vi "Raman_READ_WRITE.vi"(8 "error constant":errorcluster, 9 "Number of files to read":dbl=1.0, 11 "IR Read Dir.":string) -> (0 "error constant 2":errorcluster, 2 "averagePeaksStr":string, 3 "averagePeaks":dbl[](array[numeric]), 4 "Is SS?":bool)   [LabVIEW 2015]
panel:
  # "IR Data Read and Write"
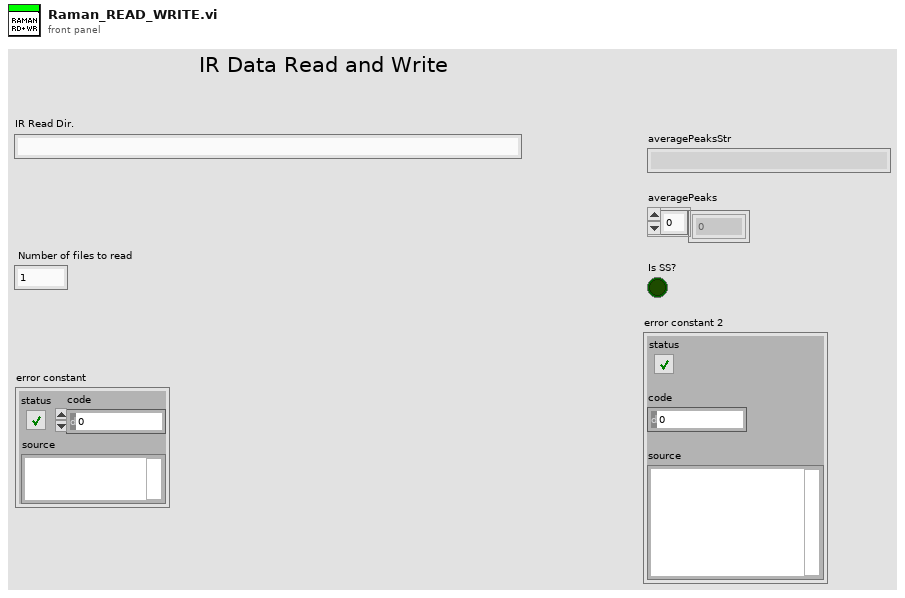
[diagram p1: front panel]
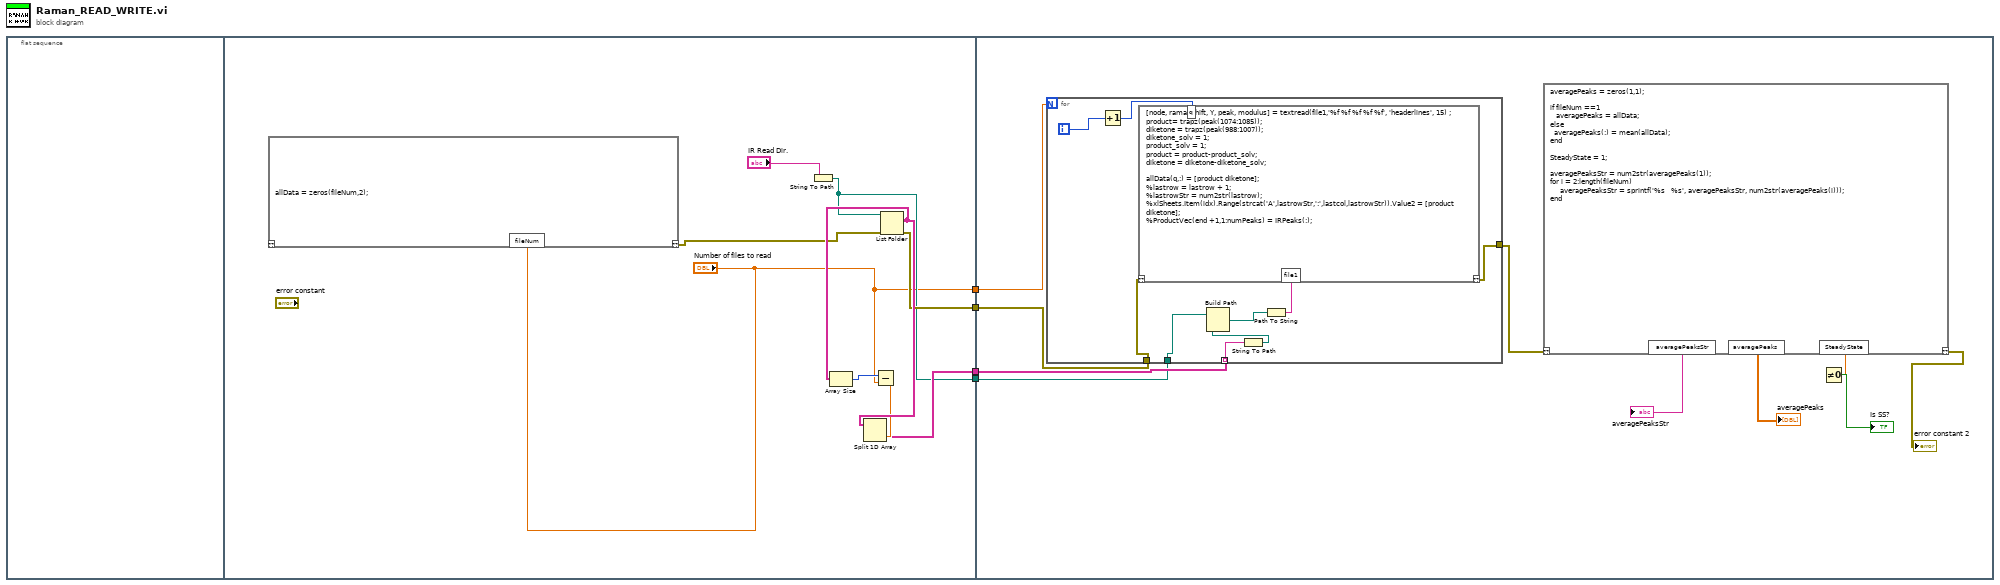
[diagram p0: block diagram]
diagram:
  n1 = flat-sequence {
    tunnel: [w8] -> w4
    tunnel: [w7] -> w3
    tunnel: [w6] -> w2
    tunnel: ["Number of files to read"] -> w1
    tunnel: w4 -> [w17]
    tunnel: w3 -> [w16]
    tunnel: w2 -> [w15]
    tunnel: w1 -> [w14]
    frame #0 {
    }
    frame #1 {
      n2 = script code="allData = zeros(fileNum,2);"("fileNum"="Number of files to read") -> ("??"=w9:errorcluster)  [unwired: 1 in]
      n3 = String To Path(string="IR Read Dir.") -> (path=w6:path)
      n4 = List Folder(path=w6, error in=w9) -> (filenames=w13:string[], error out=w8:errorcluster)  [unwired: 2 in, 2 out]
      n5 = Array Size(array=w13) -> (size(s)=w11:i32)
      n6 = Subtract(x=w11, y="Number of files to read") -> (x-y=w12:dbl)
      n7 = Split 1D Array(array=w13, index=w12) -> (second subarray=w7:string[])  [unwired: 1 out]
    }
    frame #2 {
      n8 = for {
        N: w14 -> [_]
        tunnel: w15 -> [w32]
        tunnel: w16 -> [w31] mode=indexing
        tunnel: [w26] -> w18
        tunnel: w17 -> [w25]
        i -> [w28]
        n9 = Increment(x=w28) -> (x+1=w27:i32)
        n10 = String To Path(string=w31) -> (path=w30:path)
        n11 = Build Path(base path=w32, name or relative path=w30) -> (appended path=w29:path)
        n12 = Path To String(path=w29) -> (string=w24:string)
        n13 = script code="[node, ramanshift, Y, peak, modulus] = textread(file1,'%f %f %f %f %f', 'headerlines', 15) ;\nproduct= trapz(peak(1074:1085));\ndiketone = trapz(peak(988:1007));\ndiketone_solv = 1; \nproduct_solv = 1;\nproduct = product-product_solv;\ndiketone = diketone-diketone_solv;\n\nallData(q,:) = [product diketone];\n%lastrow = lastrow + 1;\n%lastrowStr = num2str(lastrow);\n%xlSheets.Item(idx).Range(strcat('A',lastrowStr,':',lastcol,lastrowStr)).Value2 = [product diketone];\n%ProductVec(end +1,1:numPeaks) = IRPeaks(:);"("??"=w25, "q"=w27, "file1"=w24) -> ("??"=w26:errorcluster)
      }
      n14 = script code="averagePeaks = zeros(1,1);\n\nif fileNum ==1 \n   averagePeaks = allData;\nelse\n  averagePeaks(:) = mean(allData);\nend\n\nSteadyState = 1;\n\naveragePeaksStr = num2str(averagePeaks(1));\nfor i = 2:length(fileNum)\n     averagePeaksStr = sprintf('%s   %s', averagePeaksStr, num2str(averagePeaks(i)));\nend"("??"=w18) -> ("??"=→"error constant 2":errorcluster, "SteadyState"=w20:dbl, "averagePeaksStr"=→"averagePeaksStr":string, "averagePeaks"=→"averagePeaks":dbl[])
      n15 = Not Equal To 0?(x=w20) -> (x != 0?=→"Is SS?":bool)
    }
  }
